vi "UTILITY Custom VISA Name.vi"(7 "Default VISA Name":refnum<visa-resource-name>="COM3", 8 "Error In":errorcluster, 11 "Input Name (String)":string) -> (0 "Error Out":errorcluster, 3 "Name (VISA)":refnum<visa-resource-name>)   [LabVIEW 2016]
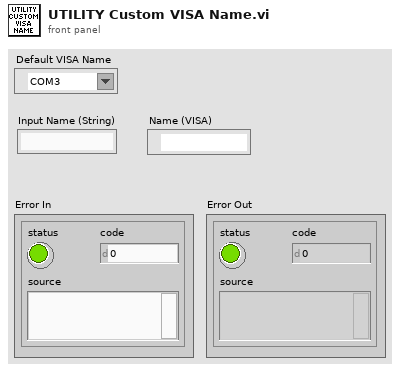
[diagram p1: front panel]
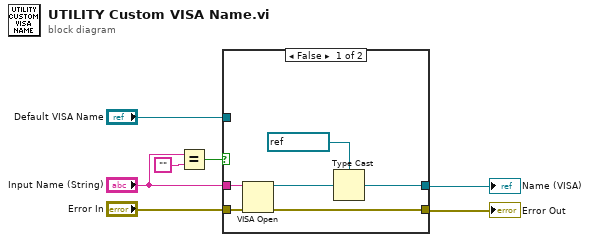
[diagram p0: block diagram]
diagram:
  n1 = Equal?(x="Input Name (String)", y="") -> (x = y?=w5:bool)
  n2 = case shown="False" w5 {
    tunnel: [w8 w14] -> w6
    tunnel: "Input Name (String)" -> [w13 _]
    tunnel: "Error In" -> [w12 w15]
    tunnel: [w11 w15] -> w2
    tunnel: "Default VISA Name" -> [_ w14]
    frame False {
      n3 = VISA Open(error in (no error)=w12, VISA resource name=w13) -> (VISA resource name=w10:refnum<visa-resource-name>, error out=w11:errorcluster)  [unwired: 3 in]
      n4 = Type Cast(type=refnum<visa-resource-name> "COM3" ("Default VISA Name 2"), x=w10) -> (*(type *) &x=w8:refnum<visa-resource-name>)
    }
    frame True {
    }
  }
  "Name (VISA)" <- w6
  "Error Out" <- w2
